vi "Method.vi"(4 "Abs_Types.lvlib:Numeric.lvclass":refnum<class "Abs_Numeric.lvclass">, 5 "Abs_Waveform.lvclass":refnum<class "Abs_Waveform.lvclass">) -> (1 "Result":refnum<class "Abs_Waveform.lvclass">)   [LabVIEW 2021, in "Add_WFM_Numeric.lvclass"]
uses:
  Add_WFM_Numeric.lvclass
  Abs_Types/Numeric/Abs_Numeric.lvclass
  Abs_Types/Waveform/Abs_Waveform.lvclass
  C:/TSA/LV_Abstract/Source/Functions/Support/Function/Two Terminal/WFM_Numeric/AbsFunc_Two Term_WFM_Numeric.lvclass
  C:/Program Files (x86)/National Instruments/LabVIEW 2021/vi.lib/TSA/Abstract Data Classes/Abs_Types/Waveform/Abs_Waveform.lvclass
  Support/Function/Two Terminal/WFM_Numeric/AbsFunc_Two Term_WFM_Numeric.lvclass/AbsFunc_Two Term_WFM_Numeric.ctl
  Support/Function/Two Terminal/WFM_Numeric/Properties/Write Abs_Waveform.lvclass.vi
  Support/Function/Two Terminal/WFM_Numeric/Properties/Write Numeric.lvclass.vi
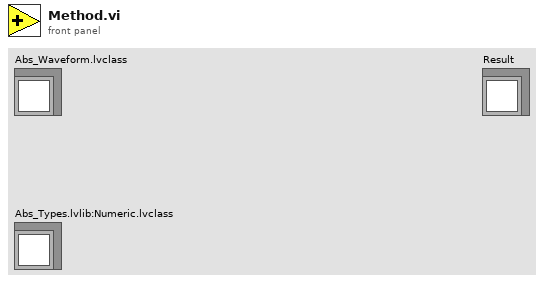
[diagram p1: front panel]
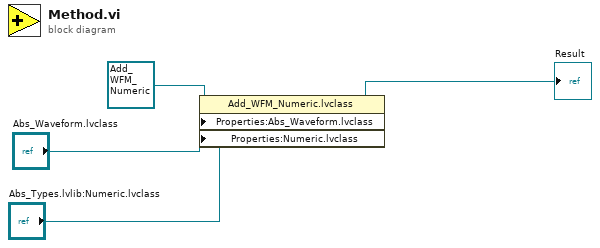
[diagram p0: block diagram]
diagram:
  n1 = property class="Add_WFM_Numeric.lvclass"(reference=refnum<class "Add_WFM_Numeric.lvclass"> refnum ("Functions.lvlib:Numeric.lvlib:Add_DBL.lvclass"), "Properties:Abs_Waveform.lvclass"="Abs_Waveform.lvclass", "Properties:Numeric.lvclass"="Abs_Types.lvlib:Numeric.lvclass") -> (reference out=→"Result":refnum<class "Add_WFM_Numeric.lvclass">)  [unwired: 1 in, 1 out]
